vi "pad Base64URL string.vi"(10 "error in (no error)":errorcluster, 11 "Base64URL string":string) -> (2 "error out":errorcluster, 3 "padded Base64 string":string)   [LabVIEW 2017]
doc: "pads a Base64URL string with \"=\" to have an a length divisible by 4."
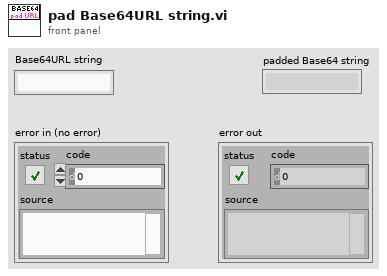
[diagram p1: front panel]
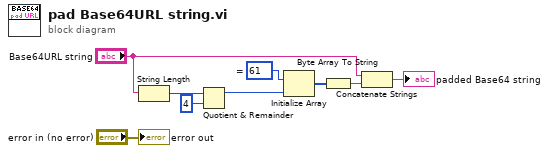
[diagram p0: block diagram]
diagram:
  w7 = u8 61  # =
  n1 = String Length(string="Base64URL string") -> (length=w9:i32)
  n2 = Quotient & Remainder(x=w9, y=4) -> (x-y*floor(x/y)=w6:i32)  [unwired: 1 out]
  n3 = Initialize Array(w7, w6) -> (w5:u8[])
  n4 = Byte Array To String(unsigned byte array=w5) -> (string=w3:string)
  n5 = Concatenate Strings("Base64URL string", w3) -> (→"padded Base64 string":string)
  "error out" <- "error in (no error)"
